vi "Set Load Parameters.vi"(8 "error in":errorcluster, 11 "3300 in":refnum<class "3300.lvclass">) -> (0 "error out":errorcluster, 3 "3300 out":refnum<class "3300.lvclass">)   [LabVIEW 2019, in "3300.lvlib" / "3300.lvclass"]
uses:
  Library/3300.lvclass
  C:/Users/Public/Documents/Development/builds/Instruments/Electronic Load.lvlibp/Library/Electronic Load.lvclass
  builds/Instruments/Electronic Load.lvlibp/Accessors/Settings/Read Mode.vi
  builds/Instruments/Electronic Load.lvlibp/Accessors/Read Active Channel.vi
  builds/Instruments/Electronic Load.lvlibp/Accessors/Settings/Read Input Level.vi
  Module Support/Access Module Limits.vi
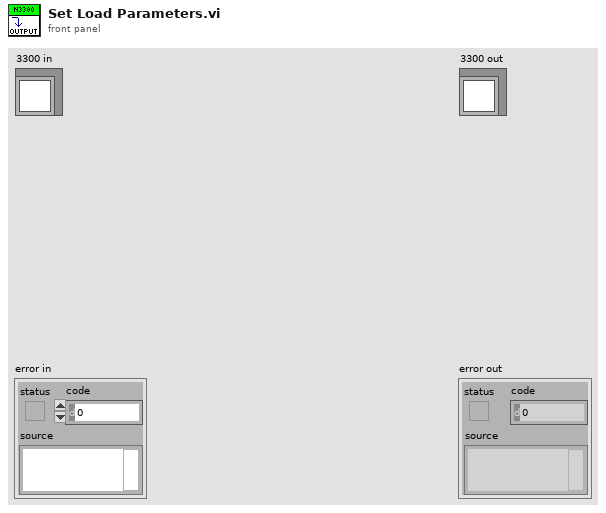
[diagram p1: front panel]
types:
  T1 = typedef "Electronic Load.lvlibp/Electronic Load.lvclass/E-Load Mode.ctl" = enum16{"Current", "Resistance", "Voltage"}
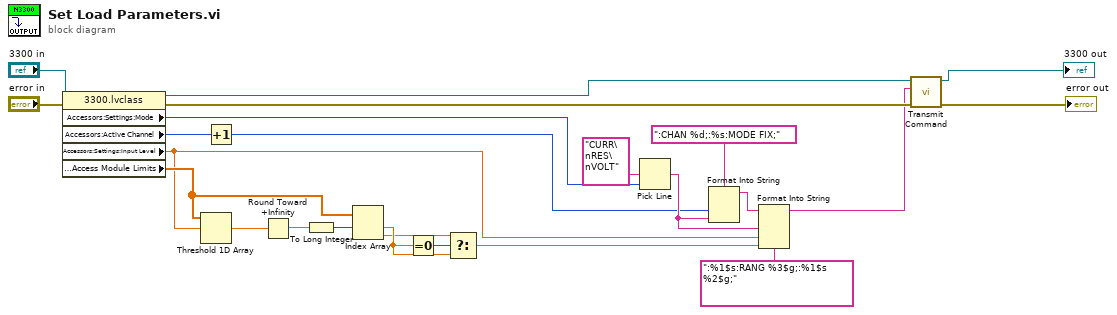
[diagram p0: block diagram]
diagram:
  n1 = property class="3300.lvclass"(reference="3300 in", error in="error in") -> (reference out=w10:refnum<class "3300.lvclass">, error out=w9:errorcluster, "Accessors:Settings:Mode"=w2:T1, "Accessors:Active Channel"=w13:u32, "Accessors:Settings:Input Level"=w11:dbl, "Private:Accessors:Access Module Limits"=w19:dbl[])
  n2 = Threshold 1D Array(2:w11, 3:w19) -> (0:w20:dbl)  [unwired: 1 in]
  n3 = Increment(x=w13) -> (x+1=w1:u32)
  n4 = Round Toward +Infinity(x=w20) -> (ceil(x): smallest int >= x=w21:dbl)
  n5 = To Long Integer(number=w21) -> (32bit integer=w22:i32)
  n6 = Index Array(array=w19, index #1=w22) -> (element #1=w17:dbl, element #2=w16:dbl)  [unwired: 1 in]
  n7 = Equal To 0?(x=w17) -> (x = 0?=w18:bool)
  n8 = Select(t=w16, s=w18, f=w17) -> (s? t:f=w12:dbl)
  n9 = Pick Line(multi-line string="CURR\nRES\nVOLT", line index=w2) -> (output string=w5:string)  [unwired: 1 in]
  n10 = Format Into String(format string=":CHAN %d;:%s:MODE FIX;", w1, w5) -> (resulting string=w3:string)  [unwired: 2 in, 1 out]
  n11 = Format Into String(format string=":%1$s:RANG %3$g;:%1$s %2$g;", initial string=w3, w5, w11, w12) -> (resulting string=w8:string)  [unwired: 1 in, 1 out]
  n12 = call "Transmit Command.vi"("error in"=w9, "Command"=w8, "3300 in"=w10) -> ("error out"=→"error out":errorcluster, "3300 out"=→"3300 out":refnum<class "3300.lvclass">)  [unwired: 7 in]
